vi "test_rm_vlc.vi"() -> ()   [LabVIEW 2023]
uses:
  <vilib>/picture/picture.llb/Draw True-Color Pixmap.vi
panel:
  out "metadata":T1
  out "pose":sgl[][](array[numeric])
  out "2D Picture":picture
  in  "stop":bool
  in  "port":u16=3800
  in  "host":string="192.168.1.7"
  in  "path in":path=path "C:/Users/jcds/Documents/GitHub/hl2ss/extensions/client_labview/hl2ss_labview/hl2ss_ulm.dll"
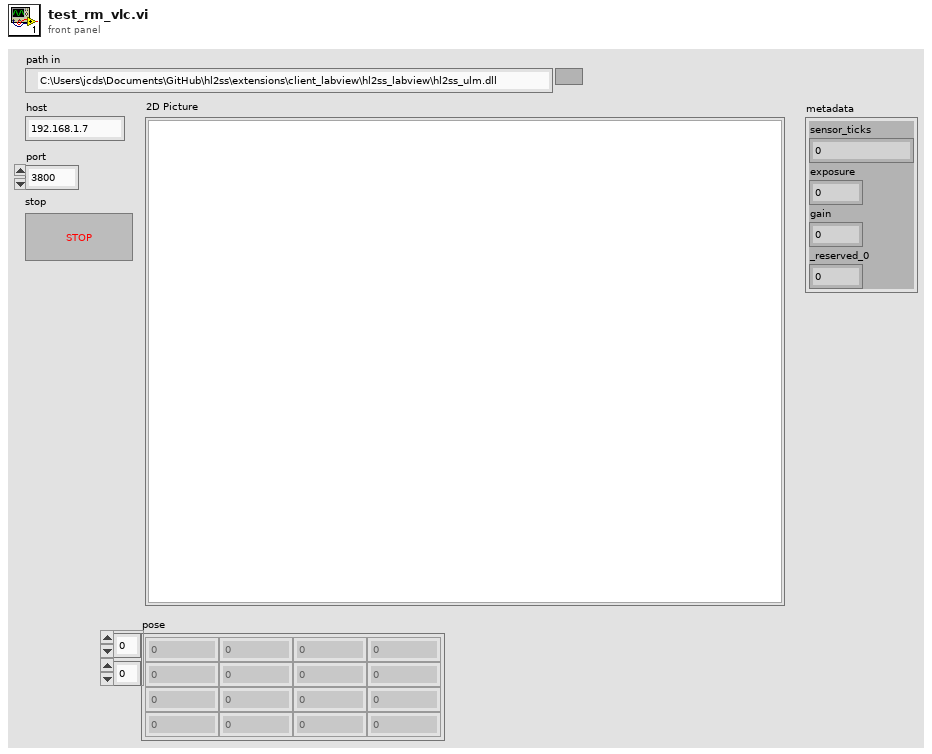
[diagram p1: front panel]
types:
  T1 = cluster{"sensor_ticks":u64, "exposure":u64, "gain":u32, "_reserved_0":u32}
  T2 = cluster{"chunk":u64, "mode":u8, "divisor":u8, "profile":u8, "level":u8, "bitrate":u32, "options_size":i64, "options_data":u64, "_reserved_0":u64}
  T3 = cluster{"frame_stamp":i64, "timestamp":u64, "payload_size":u32, "status":i32, "payload":u64, "pose":u64}
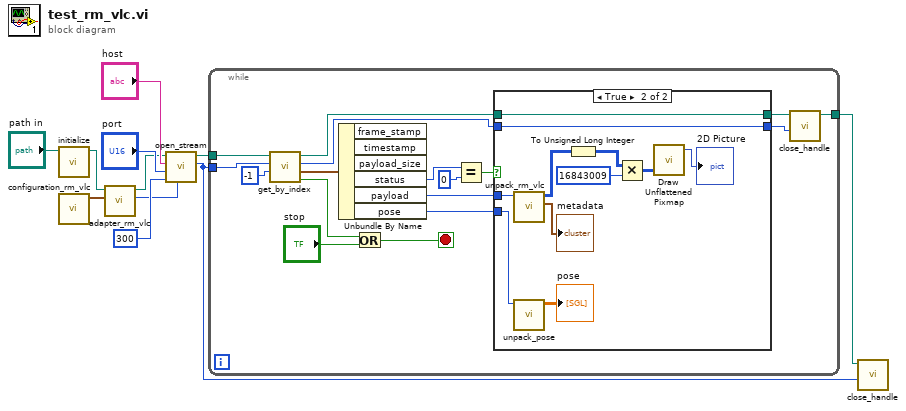
[diagram p0: block diagram]
diagram:
  n1 = call "initialize.vi"("path in"="path in") -> ("path out"=w5:path)  [unwired: 9 in, 1 out]
  n2 = call "configuration_rm_vlc.vi"() -> ("configuration_rm_vlc"=w6:T2)  [unwired: 11 in]
  n3 = call "adapter_rm_vlc.vi"("configuration_rm_vlc"=w6, "path in"=w5) -> ("configuration"=w3:u64, "path out"=w4:path)  [unwired: 8 in]
  n4 = call "open_stream.vi"("configuration"=w3, "buffer_size"=u64 300, "port"="port", "host"="host", "path in"=w4) -> ("handle"=w2:u64, "path out"=w7:path)  [unwired: 4 in, 1 out]
  n5 = while {
    tunnel: w7 -> [w28]
    tunnel: [w14] -> w1
    tunnel: w2 -> [w26]
    stop <- w19 stop-if-true
    n6 = call "get_by_index.vi"("frame_stamp"=i64 -1, "stream_handle"=w26, "path in"=w28) -> ("error"=w18:bool, "packet"=w25:T3, "packet_handle"=w20:u64, "path out"=w13:path)  [unwired: 5 in]
    n7 = Unbundle By Name(w25) -> ("status"=w24:i32, "payload"=w15:u64, "pose"=w16:u64)  [unwired: 3 out]
    n8 = Or(x=w18, y="stop") -> (x .or. y?=w19:bool)
    n9 = Equal?(x=w24, y=0) -> (x = y?=w22:bool)
    n10 = case shown="True" w22 {
      tunnel: [w30 w41] -> w21
      tunnel: w20 -> [w30 w41]
      tunnel: w16 -> [_ w39]
      tunnel: w15 -> [_ w37]
      tunnel: w13 -> [w29 w40]
      tunnel: [w29 w40] -> w12
      frame False {
      }
      frame True {
        n11 = call "unpack_rm_vlc.vi"("payload"=w37) -> ("rm_vlc_metadata"=→"metadata":T1, "image"=w34:u8[][])  [unwired: 8 in, 1 out]
        n12 = call "unpack_pose.vi"("pose"=w39) -> ("pose"=→"pose":sgl[][])  [unwired: 9 in, 1 out]
        n13 = To Unsigned Long Integer(number=w34) -> (unsigned 32bit integer=w33:u32[][])
        n14 = Multiply(x=w33, y=u32 16843009) -> (x*y=w31:u32[][])
        n15 = call-poly <vilib>:"Draw Unflattened Pixmap.vi"("data (RGB format)"=w31) -> ("new picture"=→"2D Picture":picture)  [unwired: 8 in]
      }
    }
    n16 = call "close_handle.vi"("handle"=w21, "path in"=w12) -> ("path out"=w14:path)  [unwired: 9 in]
  }
  n17 = call "close_handle.vi"("handle"=w2, "path in"=w1) -> ()  [unwired: 9 in, 1 out]
